vi "Motor_Close.vi"() -> ()   [LabVIEW 2009, in "Motor.lvlib"]
uses:
  Motor.lvlib
  PWM/PWM_Name.ctl
  PWM.lvlib
  FPGA.lvlib
panel:
  in  "error in":errorcluster
  out "error out":errorcluster
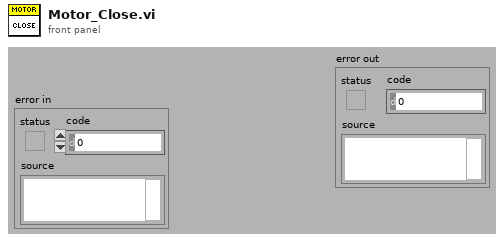
[diagram p1: front panel]
types:
  T1 = typedef "PWM.lvlib/PWM_Name.ctl" = u16
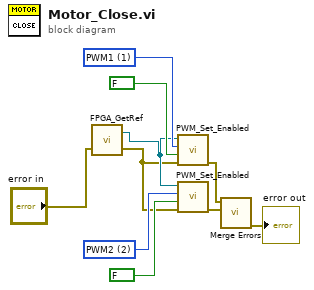
[diagram p0: block diagram]
diagram:
  w6 = T1 2 items=["Invalid"=0, "PWM1"=1, "PWM2"=2, "PWM9"=9, "PWM10"=10] ("PWM_in")
  w7 = T1 1 items=["Invalid"=0, "PWM1"=1, "PWM2"=2, "PWM9"=9, "PWM10"=10] ("PWM_in")
  n1 = call "FPGA_GetRef.vi"("error in (no error)"="error in") -> ("error out"=w1:errorcluster, "FPGA_Ref"=w3:refnum<k20>)  [unwired: 1 in]
  n2 = call "PWM_Set_Enabled.vi"("error in"=w1, "Enable"=FALSE, "PWM_in"=w7, "FPGA_Ref_in"=w3) -> ("error out"=w9:errorcluster)  [unwired: 5 in, 2 out]
  n3 = call "PWM_Set_Enabled.vi"("error in"=w1, "Enable"=FALSE, "PWM_in"=w6, "FPGA_Ref_in"=w3) -> ("error out"=w8:errorcluster)  [unwired: 5 in, 2 out]
  n4 = call <vilib>:"Merge Errors.vi"("error in 2 (no error)"=w8, "error in 1 (no error)"=w9) -> ("error out"=→"error out":errorcluster)  [unwired: 5 in]
